vi "Get Schedules for the Process.vi"(8 "error in (no error)":errorcluster, 10 "Process ID":string, 11 "Tamer in":refnum<class "Tamer.lvclass">=refnum) -> (0 "error out":errorcluster, 1 "Schedules":refnum<class "Schedule.lvclass">[](array[class]), 2 "Sync. Mask":T1[](array[typedef]), 3 "Tamer out":refnum<class "Tamer.lvclass">)   [LabVIEW 2020, in "CIRCUS_uServices.lvlib" / "Tamer.lvlib" / "Tamer.lvclass"]
doc: "Get list of schedules and sync mask for Monkeys for specified process"
uses:
  Tamer.lvclass
  Run Utilities/Schedule/Schedule.lvclass
  Run Utilities/TypeDefs/Synchronize FPGA Cluster.ctl
  Run Utilities/Run Utilities.lvlib
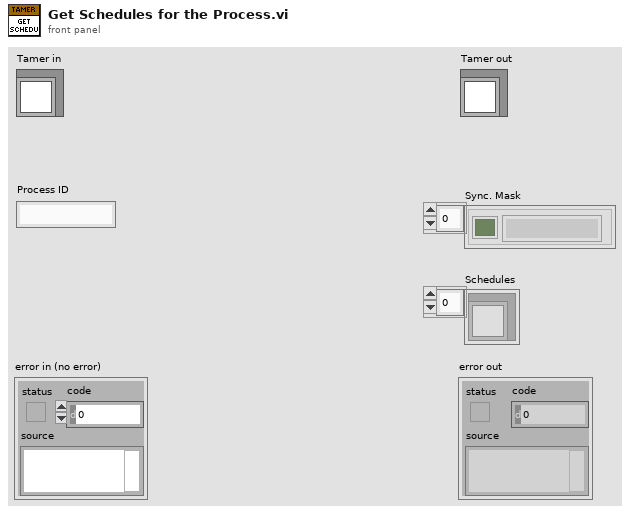
[diagram p1: front panel]
types:
  T1 = typedef "CIRCUS_uServices.lvlib/Run Utilities.lvlib/Synchronize FPGA Cluster.ctl" = cluster{"Status":bool, "FPGA Name":string}
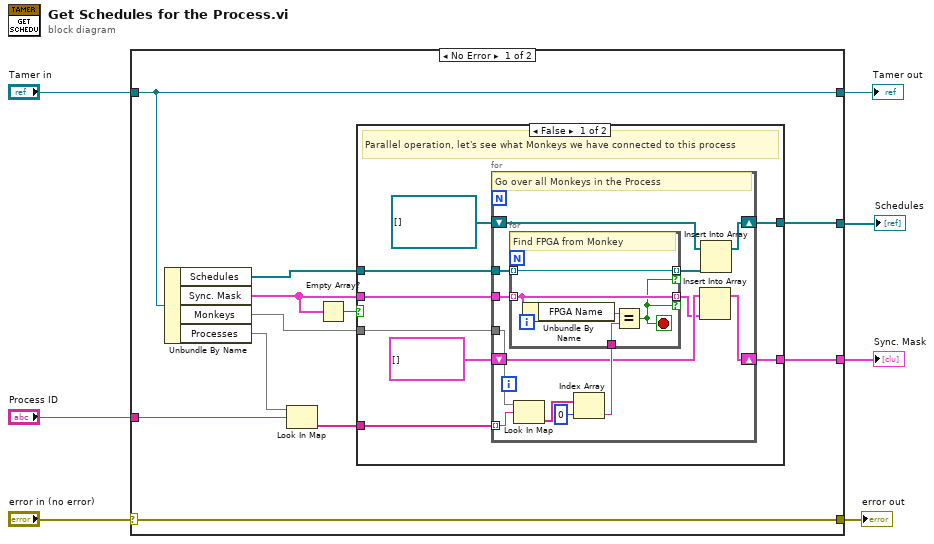
[diagram p0: block diagram]
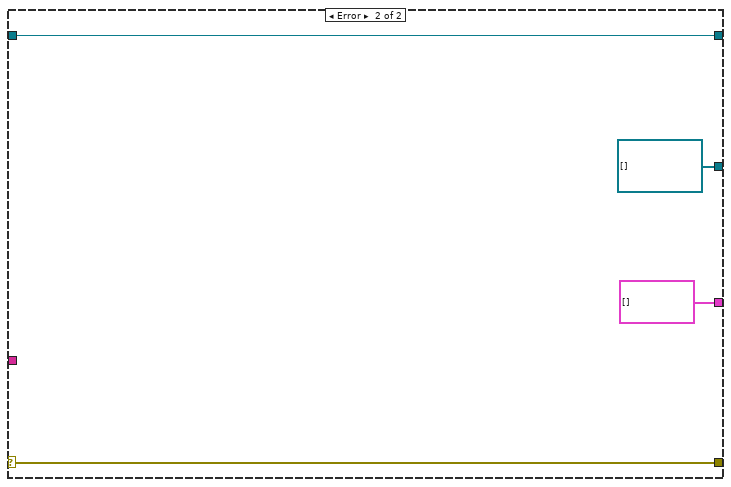
[diagram p3: hidden frame]
diagram:
  n1 = case shown="No Error" "error in (no error)" {
    selector: "error in (no error)" -> [w18 w50]
    tunnel: [w18 w50] -> w6
    tunnel: [w11 w49] -> w4
    tunnel: "Tamer in" -> [w11 w49]
    tunnel: "Process ID" -> [w17 _]
    tunnel: [w15 refnum<class "Schedule.lvclass">[] [] ("Schedules")] -> w2
    tunnel: [w13 T1[] [] ("Sync. Mask")] -> w1
    frame No Error {
      n2 = Unbundle By Name(w11) -> ("Schedules"=w10:refnum<class "Schedule.lvclass">[], "Sync. Mask"=w14:T1[], "Monkeys"=w8:map{string, string[]}, "Processes"=w9:map{string, string[]})
      n3 = Look In Map(map=w9, key=w17) -> (value=w12:string[])  [unwired: 1 in, 1 out]
      n4 = Empty Array?(array=w14) -> (empty?=w16:bool)
      n5 = case shown="False" w16 {
        tunnel: w10 -> [w26 w46]
        tunnel: [w19 w46] -> w15
        tunnel: w14 -> [w25 w45]
        tunnel: [w20 w45] -> w13
        tunnel: w12 -> [w24 _]
        tunnel: w8 -> [w23 _]
        frame False {
          # "Parallel operation, let's see what Monkeys we have connected to this process"
          n6 = for {
            tunnel: w26 -> [w38]
            tunnel: w25 -> [w39]
            tunnel: w24 -> [w36] mode=indexing
            tunnel: w23 -> [w37]
            shift-right: [w30] -> w19
            shift-left: refnum<class "Schedule.lvclass">[] [] -> [w31]
            shift-right: [w29] -> w20
            shift-left: T1[] [] -> [w28]
            # "Go over all Monkeys in the Process"
            n7 = Look In Map(map=w37, key=w36) -> (value=w35:string[])  [unwired: 1 in, 1 out]
            n8 = Index Array(array=w35, index=0) -> (element=w33:string)
            n9 = for {
              tunnel: w39 -> [w42] mode=indexing
              tunnel: w38 -> [w41] mode=indexing
              tunnel: w33 -> [w44]
              tunnel: [w42] -> w27 mode=indexing if=w40
              tunnel: [w41] -> w32 mode=indexing if=w40
              stop <- w40 stop-if-true
              # "Find FPGA from Monkey"
              n10 = Unbundle By Name(w42) -> ("FPGA Name"=w43:string)
              n11 = Equal?(x=w43, y=w44) -> (x = y?=w40:bool)
            }
            n12 = Insert Into Array(array=w28, new element=w27) -> (w29:T1[])  [unwired: 1 in]
            n13 = Insert Into Array(array=w31, new element=w32) -> (w30:refnum<class "Schedule.lvclass">[])  [unwired: 1 in]
          }
        }
        frame True {
          # "No sync mask, this is standard operation. There is one Monkey and one schedule"
        }
      }
    }
    frame Error {
    }
  }
  "error out" <- w6
  "Tamer out" <- w4
  "Schedules" <- w2
  "Sync. Mask" <- w1
